vi "Attendance_Panel.vi"(8 "error in (no error)":errorcluster, 11 "PanelController":refnum<class "MemberPanel.lvclass">) -> (0 "error out":errorcluster, 3 "CalAttendance out":refnum<class "CalAttendance.lvclass">)   [LabVIEW 2015, in "Admin_Actor.lvlib"]
uses:
  Admin_Actor.lvlib
  CalAttendance/Type Definitions/NumOfAttendace.ctl
  CalAttendance/Type Definitions/Sign_Attendance.ctl
  CalAttendance/CalAttendance.lvclass
  Member_Actor/MemberPanel/MemberPanel.lvclass
  CalAttendance/Type Definitions/Main Ctls and VI Refs.ctl
  <vilib>/Utility/error.llb/Error Cluster From Error Code.vi
  Setting/g_setting.vi
  <vilib>/ErrorRing/Error Ring.xnode
panel:
  in  "RenewGroup":bool
  out "Sign_Attendance":T1
  out "Num_Attendance":T2
  in  "周次":i32
  in  "组别":string(combo)
  in  "姓名":string(combo)
  in  "Path":path
  in  "Stop":bool
  in  "Save":bool
  in  "Import":bool
  in  "schedule":cluster{"BackGround":u32, "Reason":string}[][](array[cluster])
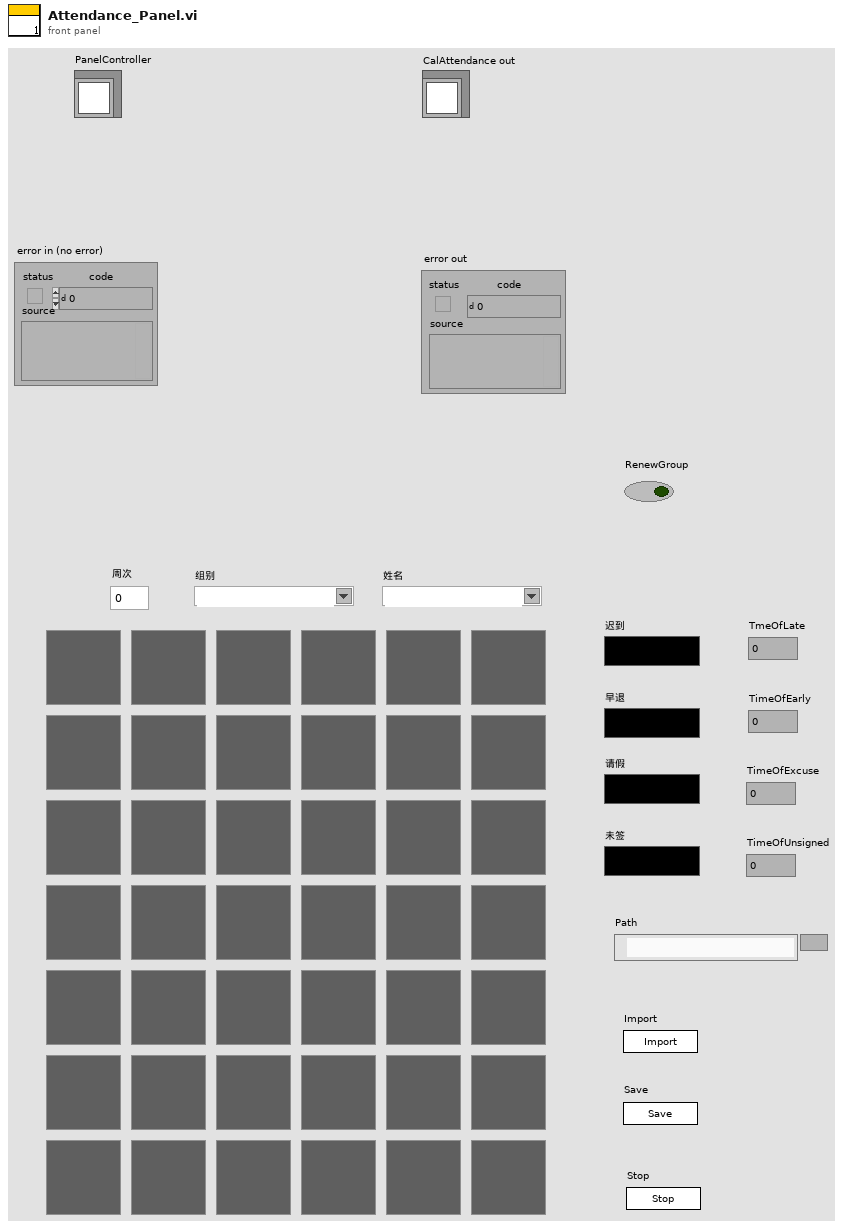
[diagram p1: front panel]
types:
  T1 = typedef "CalAttendance.lvclass/Sign_Attendance.ctl" = cluster{"早退":u32, "迟到":u32, "请假":u32, "未签":u32}
  T2 = typedef "CalAttendance.lvclass/NumOfAttendace.ctl" = cluster{"TmeOfLate":i32, "TimeOfEarly":i32, "TimeOfExcuse":i32, "TimeOfUnsigned":i32}
  T3 = typedef "CalAttendance.lvclass/Main Ctls and VI Refs.ctl" = cluster{"Num_Attendance":refnum<vi>, "Sign_Attendance":refnum<vi>, "Path":refnum<vi>, "周次":refnum<vi>, "姓名":refnum<vi>, "组别":refnum<vi>, "schedule":refnum<vi>, "VI Refnum":refnum<vi>}
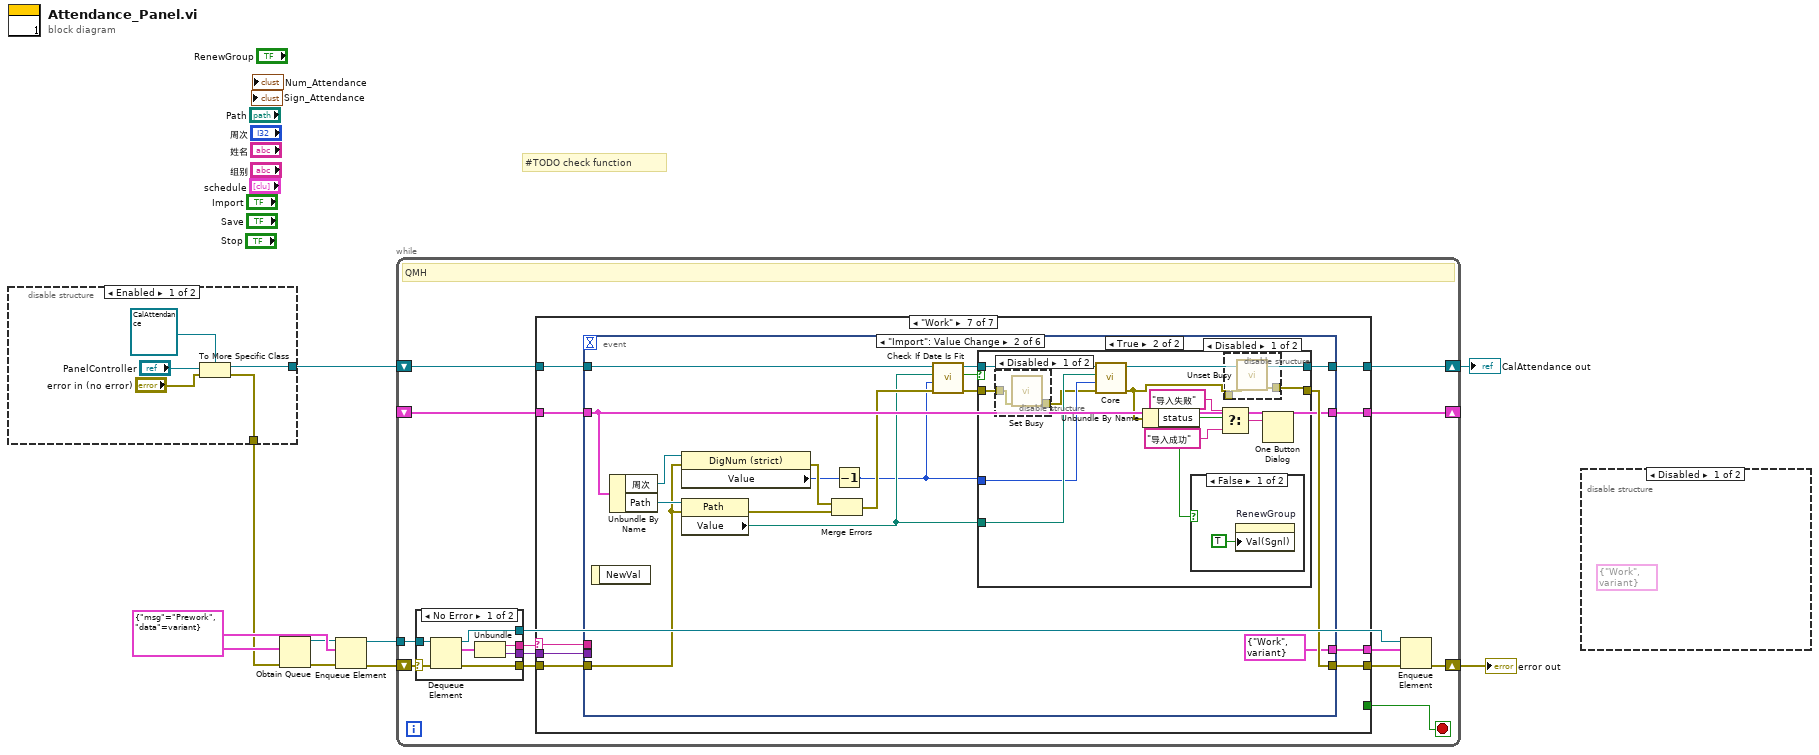
[diagram p0: block diagram]
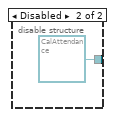
[diagram p2: hidden frame]
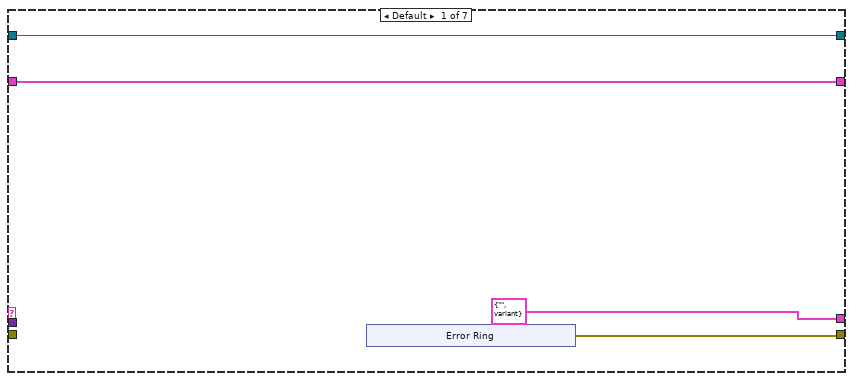
[diagram p4: hidden frame]
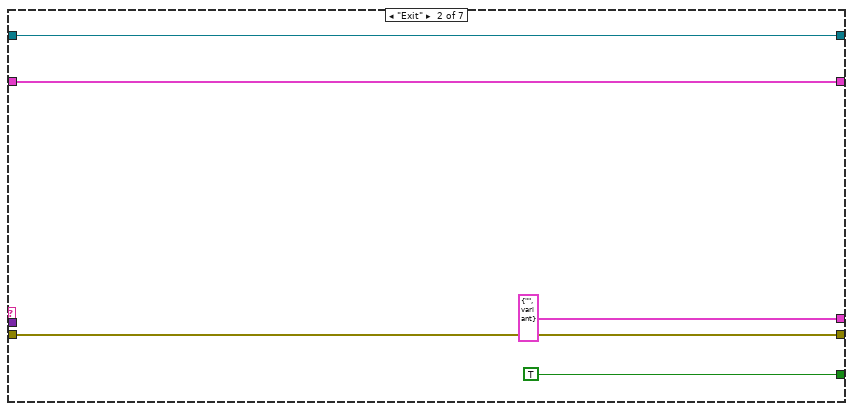
[diagram p5: hidden frame]
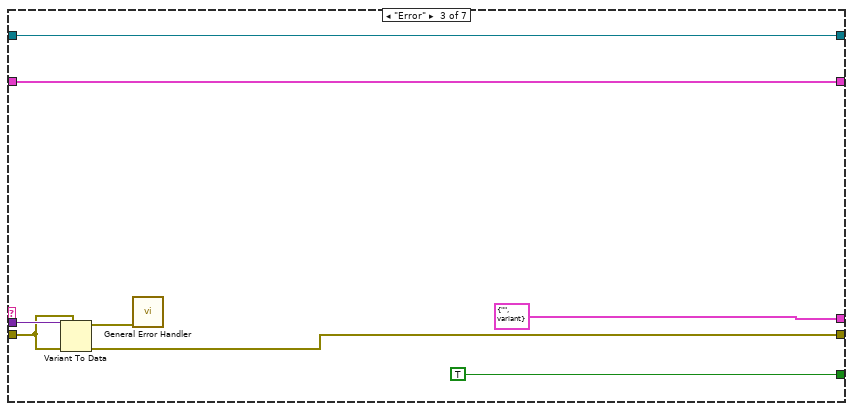
[diagram p6: hidden frame]
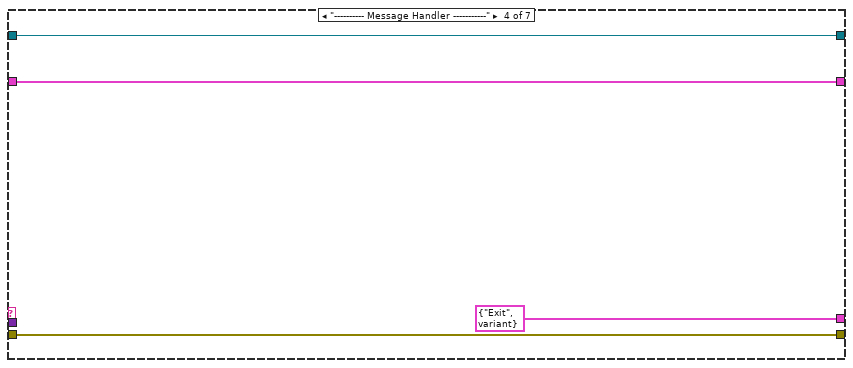
[diagram p7: hidden frame]
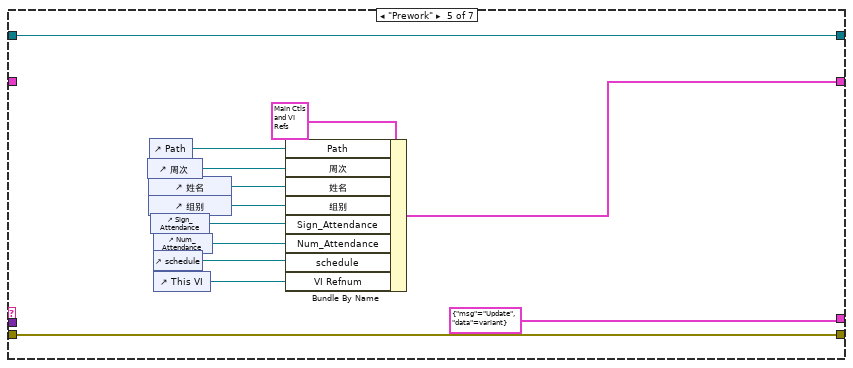
[diagram p8: hidden frame]
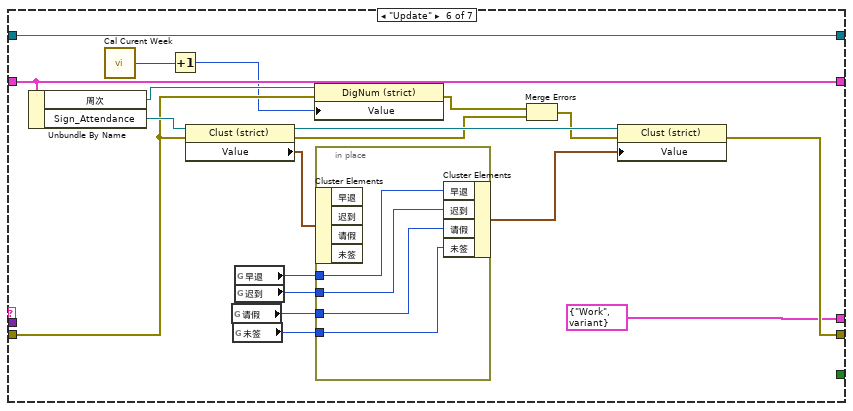
[diagram p9: hidden frame]
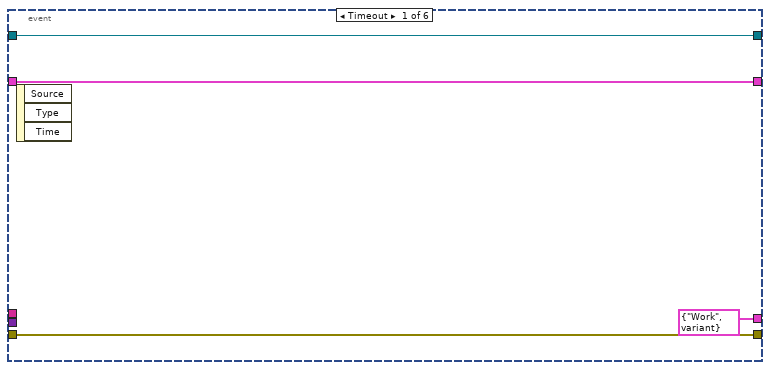
[diagram p10: hidden frame]
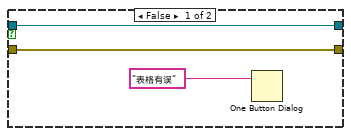
[diagram p11: hidden frame]
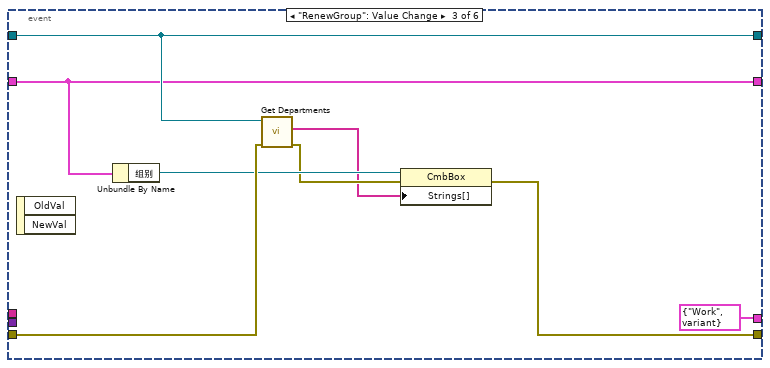
[diagram p15: hidden frame]
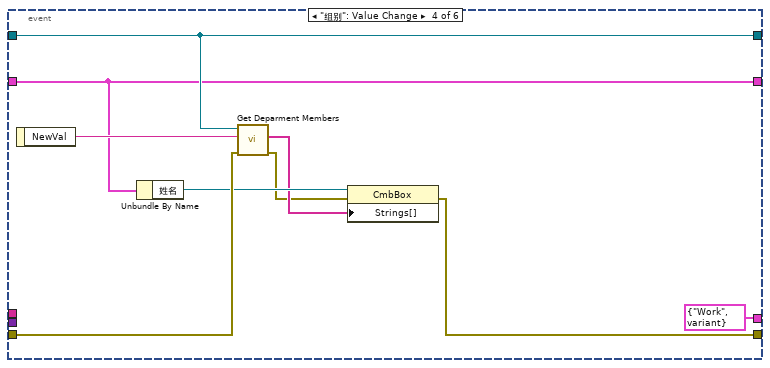
[diagram p16: hidden frame]
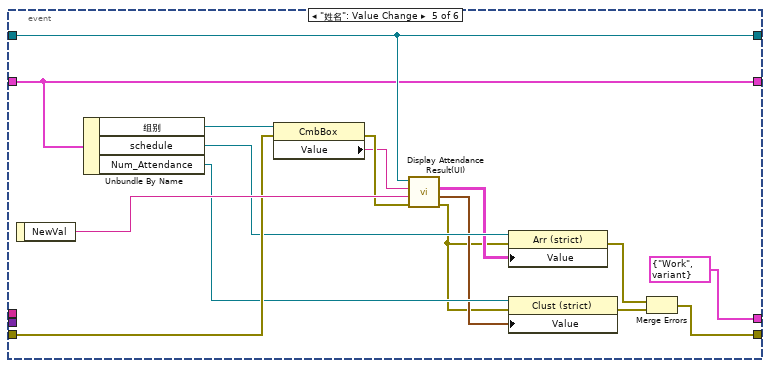
[diagram p17: hidden frame]
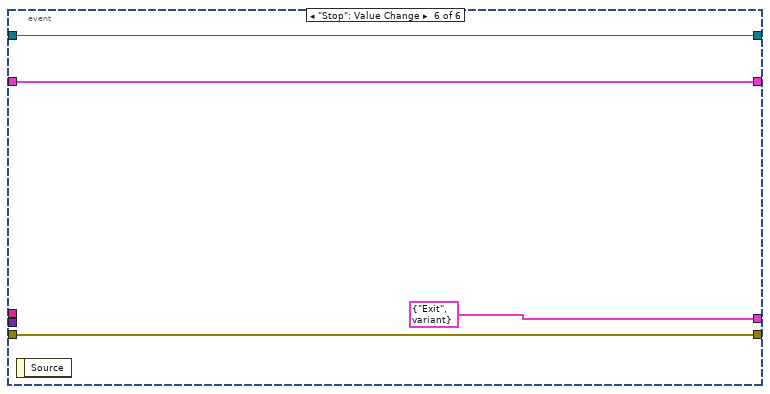
[diagram p18: hidden frame]
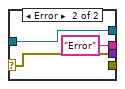
[diagram p19: hidden frame]
diagram:
  w7 = cluster{"msg":string, "data":variant} {"msg"="Prework", "data"=variant}
  # "#TODO check function"
  n1 = disable-structure shown="Enabled" {
    disable-tunnel: [w12 refnum<class "CalAttendance.lvclass"> refnum ("CalAttendance")] -> w2
    disable-tunnel: [w10 _] -> w1
    frame Enabled {
      n2 = To More Specific Class(target class=refnum<class "CalAttendance.lvclass"> refnum ("CalAttendance"), reference="PanelController", error in="error in (no error)") -> (specific class reference=w12:refnum<class "CalAttendance.lvclass">, error out=w10:errorcluster)
    }
    frame Disabled {
    }
  }
  n3 = Obtain Queue(element data type=w7, error in (no error)=w1) -> (queue out=w5:refnum<queue>, error out=w6:errorcluster)  [unwired: 3 in, 1 out]
  n4 = Enqueue Element(queue=w5, element=w7, error in (no error)=w6) -> (queue out=w8:refnum<queue>, error out=w9:errorcluster)  [unwired: 1 in, 1 out]
  n5 = while {
    tunnel: w8 -> [w28]
    shift-right: [w23] -> w3
    shift-left: w9 -> [w29]
    shift-right: [w19] -> _
    shift-left: _ -> [w18]
    shift-right: [w17] -> w4
    shift-left: w2 -> [w16]
    stop <- w20 stop-if-true
    # "QMH"
    n6 = case shown="No Error" w29 {
      selector: w29 -> [w184 w188]
      tunnel: w28 -> [w185 w186]
      tunnel: [w183 _] -> w27
      tunnel: [w181 "Error" ("msg")] -> w26
      tunnel: [w180 w188] -> w25
      tunnel: [w179 w186] -> w22
      frame No Error {
        n7 = Dequeue Element(queue=w185, error in (no error)=w184) -> (queue out=w179:refnum<queue>, element=w182:cluster{"msg":string, "data":variant}, error out=w183:errorcluster)  [unwired: 1 in, 1 out]
        n8 = Unbundle(w182) -> ("msg"=w181:string, "data"=w180:variant)
      }
      frame Error {
      }
    }
    n9 = case shown="\"Work\"" w26 {
      selector: w26 -> [_ _ _ _ _ _ w98]
      tunnel: w27 -> [_ w43 w50 w55 w67 w74 w100]
      tunnel: w25 -> [_ _ w51 _ _ _ w99]
      tunnel: [w33 w43 w48 w55 w67 w81 w97] -> w24
      tunnel: [cluster{"msg":string, "data":variant} {"msg"="", "data"=variant} cluster{"msg":string, "data":variant} {"msg"="", "data"=variant} cluster{"msg":string, "data":variant} {"msg"="", "data"=variant} cluster{"msg":string, "data":variant} {"msg"="Exit", "data"=variant} cluster{"msg":string, "data":variant} {"msg"="Update", "data"=variant} cluster{"msg":string, "data":variant} {"msg"="Work", "data"=variant} w96] -> w21
      tunnel: [_ TRUE TRUE _ _ _ _] -> w20
      tunnel: [w30 w39 w44 w52 w65 w86 w92] -> w19
      tunnel: w18 -> [w30 w39 w44 w52 _ w86 w94]
      tunnel: [w31 w40 w45 w53 w56 w87 w93] -> w17
      tunnel: w16 -> [w31 w40 w45 w53 w56 w87 w95]
      frame Default {
        n10 = xnode ("Error Ring")() -> ("error out"=w33:errorcluster)
      }
      frame "Exit" {
      }
      frame "Error" {
        n11 = Variant To Data(error in=w50, type=w50, Variant=w51) -> (data=w49:errorcluster, error out=w48:errorcluster)
        n12 = call <vilib>:"General Error Handler.vi"("error in (no error)"=w49) -> ()  [unwired: 10 in, 5 out]
      }
      frame "---------- Message Handler -----------" {
      }
      frame "Prework" {
        n13 = control-ref of="周次"() -> (w64:refnum<vi>)
        n14 = control-ref of="姓名"() -> (w63:refnum<vi>)
        n15 = control-ref of="组别"() -> (w62:refnum<vi>)
        n16 = control-ref of="Path"() -> (w61:refnum<vi>)
        n17 = control-ref of="Sign_Attendance"() -> (w60:refnum<vi>)
        n18 = control-ref of="Num_Attendance"() -> (w59:refnum<vi>)
        n19 = control-ref of="schedule"() -> (w58:refnum<vi>)
        n20 = control-ref of="This VI"() -> (w57:refnum<vi>)
        n21 = Bundle By Name(cluster=T3 {"Num_Attendance"=refnum, "Sign_Attendance"=refnum, "Path"=refnum, "周次"=refnum, "姓名"=refnum, "组别"=refnum, "schedule"=refnum, "VI Refnum"=refnum} ("Refs"), "Path"=w61, "周次"=w64, "姓名"=w63, "组别"=w62, "Sign_Attendance"=w60, "Num_Attendance"=w59, "schedule"=w58, "VI Refnum"=w57) -> (w65:T3)
      }
      frame "Update" {
        n22 = Unbundle By Name(w86) -> ("周次"=w75:refnum<vi>, "Sign_Attendance"=w85:refnum<vi>)
        n23 = call "Cal Curent Week.vi"() -> ("CurWeek(0)"=w70:i32)
        n24 = Increment(x=w70) -> (x+1=w69:i32)
        n25 = property class="Clust (strict)"(reference=w85, error in=w74) -> (reference out=w83:refnum<vi>, error out=w72:errorcluster, "Value"=w84:cluster{"早退":u32, "迟到":u32, "请假":u32, "未签":u32})
        n26 = global read "g_setting.vi" "请假"() -> (w77:u32)
        n27 = global read "g_setting.vi" "未签"() -> (w76:u32)
        n28 = global read "g_setting.vi" "早退"() -> (w79:u32)
        n29 = global read "g_setting.vi" "迟到"() -> (w78:u32)
        n30 = property class="DigNum (strict)"(reference=w75, error in=w74, "Value"=w69) -> (error out=w73:errorcluster)  [unwired: 1 out]
        n31 = in-place {
          in-place-border: w79 -> [w91]
          in-place-border: w78 -> [w90]
          in-place-border: w77 -> [w89]
          in-place-border: w76 -> [w88]
          n32 = in-place-cluster #1(w84) -> ()  [unwired: 4 out]
          n33 = in-place-cluster #1("早退"=w91, "迟到"=w90, "请假"=w89, "未签"=w88) -> (w82:cluster{"早退":u32, "迟到":u32, "请假":u32, "未签":u32})
        }
        n34 = Merge Errors(w73, w72) -> (w71:errorcluster)
        n35 = property class="Clust (strict)"(reference=w83, error in=w71, "Value"=w82) -> (error out=w81:errorcluster)  [unwired: 1 out]
      }
      frame "Work" {
        n36 = event shown="[1] \"Import\": Value Change" {
          selector: _ -> [_ _ _ _ _ _]
          dyn-events: _ -> [_ _ _ _ _ _]
          timeout: _ -> [_ _ _ _ _ _]
          tunnel: w100 -> [w104 w119 w147 w156 w170 w178]
          tunnel: w99 -> [_ _ _ _ _ _]
          tunnel: w98 -> [_ _ _ _ _ _]
          tunnel: [w104 w116 w143 w151 w160 w178] -> w97
          tunnel: [cluster{"msg":string, "data":variant} {"msg"="Work", "data"=variant} cluster{"msg":string, "data":variant} {"msg"="Work", "data"=variant} cluster{"msg":string, "data":variant} {"msg"="Work", "data"=variant} cluster{"msg":string, "data":variant} {"msg"="Work", "data"=variant} cluster{"msg":string, "data":variant} {"msg"="Work", "data"=variant} cluster{"msg":string, "data":variant} {"msg"="Exit", "data"=variant}] -> w96
          tunnel: w95 -> [w102 w113 w149 w158 w174 w176]
          tunnel: w94 -> [w101 w114 w148 w155 w172 w175]
          tunnel: [w102 w115 w149 w158 w174 w176] -> w93
          tunnel: [w101 w114 w148 w155 w172 w175] -> w92
          event Timeout {
            n37 = event-data() -> ()  [unwired: 1 in, 3 out]
          }
          event "Import": Value Change {
            n38 = event-data() -> ()  [unwired: 1 in, 1 out]
            n39 = Unbundle By Name(w114) -> ("周次"=w120:refnum<vi>, "Path"=w121:refnum<vi>)
            n40 = property class="DigNum (strict)"(reference=w120, error in=w119) -> (error out=w118:errorcluster, "Value"=w106:i32)  [unwired: 1 out]
            n41 = property class="Path"(reference=w121, error in=w119) -> (error out=w117:errorcluster, "Value"=w111:path)  [unwired: 1 out]
            n42 = Merge Errors(w118, w117) -> (w112:errorcluster)
            n43 = Decrement(x=w106) -> (x-1=w105:i32)
            n44 = call "Check If Date Is Fit.vi"("error in (no error)"=w112, "CurWeek(0)"=w105, "Path"=w111, "CalAttendance in"=w113) -> ("error out"=w110:errorcluster, "Fit(False)"=w108:bool, "CalAttendance out"=w109:refnum<class "CalAttendance.lvclass">)  [unwired: 5 in]
            n45 = case shown="True" w108 {
              tunnel: [w123 w127] -> w116
              tunnel: [w124 w136] -> w115
              tunnel: w111 -> [_ w135]
              tunnel: w105 -> [_ w134]
              tunnel: w110 -> [w123 w129]
              tunnel: w109 -> [w124 w133]
              frame False {
                n46 = One Button Dialog(message="表格有误") -> ()  [unwired: 1 in, 1 out]
              }
              frame True {
                n47 = disable-structure shown="Disabled" {
                  disable-tunnel: w129 -> [w140 _]
                  disable-tunnel: [w139 _] -> w128
                  frame Disabled {
                    n48 = call <vilib>:"Set Busy.vi"("error in (no error)"=w140) -> ("error out"=w139:errorcluster)  [unwired: 9 in, 1 out]
                  }
                  frame Enabled {
                  }
                }
                n49 = call "Core.vi"("error in (no error)"=w128, "CurWeek(0)"=w134, "ExcusePath"=w135, "CalAttendance in"=w133) -> ("error out"=w126:errorcluster, "CalAttendance out"=w136:refnum<class "CalAttendance.lvclass">)  [unwired: 6 in]
                n50 = Unbundle By Name(w126) -> ("status"=w125:bool)
                n51 = case shown="False" w125 {
                  frame False {
                    n52 = property on="RenewGroup" class="Bool (strict)"("Val(Sgnl)"=TRUE ("Value (Signaling)")) -> ()  [unwired: 2 in, 2 out]
                  }
                  frame True {
                  }
                }
                n53 = Select(t="导入失败", s=w125, f="导入成功") -> (s? t:f=w130:string)
                n54 = disable-structure shown="Disabled" {
                  disable-tunnel: [w138 _] -> w127
                  disable-tunnel: w126 -> [w137 _]
                  frame Disabled {
                    n55 = call <vilib>:"Unset Busy.vi"("error in (no error)"=w137) -> ("error out"=w138:errorcluster)  [unwired: 10 in]
                  }
                  frame Enabled {
                  }
                }
                n56 = One Button Dialog(message=w130) -> ()  [unwired: 1 in, 1 out]
              }
            }
          }
          event "RenewGroup": Value Change {
            n57 = event-data() -> ()  [unwired: 1 in, 2 out]
            n58 = Unbundle By Name(w148) -> ("组别"=w146:refnum<vi>)
            n59 = call "Get Departments.vi"("error in (no error)"=w147, "CalAttendance in"=w149) -> ("error out"=w145:errorcluster, "Departments(\"\")"=w144:string[])  [unwired: 7 in, 1 out]
            n60 = property class="CmbBox"(reference=w146, error in=w145, "Strings[]"=w144) -> (error out=w143:errorcluster)  [unwired: 1 out]
          }
          event "组别": Value Change {
            n61 = event-data() -> ("NewVal"=w157:string)  [unwired: 1 in]
            n62 = Unbundle By Name(w155) -> ("姓名"=w154:refnum<vi>)
            n63 = call "Get Deparment Members.vi"("error in (no error)"=w156, "Department(\"\")"=w157, "CalAttendance in"=w158) -> ("error out"=w152:errorcluster, "Names(\"\")"=w153:string[])  [unwired: 6 in, 1 out]
            n64 = property class="CmbBox"(reference=w154, error in=w152, "Strings[]"=w153) -> (error out=w151:errorcluster)  [unwired: 1 out]
          }
          event "姓名": Value Change {
            n65 = event-data() -> ("NewVal"=w173:string)  [unwired: 1 in]
            n66 = Unbundle By Name(w172) -> ("组别"=w171:refnum<vi>, "schedule"=w167:refnum<vi>, "Num_Attendance"=w165:refnum<vi>)
            n67 = property class="CmbBox"(reference=w171, error in=w170) -> (error out=w169:errorcluster, "Value"=w168:string)  [unwired: 1 out]
            n68 = call "Display Attendance Result(UI).vi"("error in (no error)"=w169, "Name(\"\")"=w173, "Department(\"\")"=w168, "CalAttendance in"=w174) -> ("error out"=w163:errorcluster, "NumOfAttendance"=w164:T2, "Res_Attendance"=w166:cluster{"BackGround":u32, "Reason":string}[][])  [unwired: 4 in, 1 out]
            n69 = property class="Arr (strict)"(reference=w167, error in=w163, "Value"=w166) -> (error out=w162:errorcluster)  [unwired: 1 out]
            n70 = property class="Clust (strict)"(reference=w165, error in=w163, "Value"=w164) -> (error out=w161:errorcluster)  [unwired: 1 out]
            n71 = Merge Errors(w162, w161) -> (w160:errorcluster)
          }
          event "Stop": Value Change {
            n72 = event-data() -> ()  [unwired: 1 in, 1 out]
          }
        }
      }
    }
    n73 = Enqueue Element(queue=w22, element=w21, error in (no error)=w24) -> (error out=w23:errorcluster)  [unwired: 1 in, 2 out]
  }
  "CalAttendance out" <- w4
  "error out" <- w3
  n74 = disable-structure shown="Disabled" {
    frame Disabled {
      (unwired) cluster{"msg":string, "data":variant} {"msg"="Work", "data"=variant}
    }
    frame Enabled {
    }
  }
